vi "FPGA_I2C_Globals.vi"() -> ()   [LabVIEW 2020]
doc: "Stores configuration information for the I2C engine to be used by the top-level FPGA VI."
uses:
  Controls/FPGA I2C_Cmd.ctl
panel:
  in  "I2C_Address":u16
  in  "I2C_Bytes to Write":u16=1
  in  "I2C_Bytes to Read":u16=1
  in  "I2C_Wait Time/2":u32
  in  "I2C_Wait Time":u32
  in  "I2C_Cmd":T1=enum."Configure"
  out "I2C_Done":bool
  out "I2C_Start":bool
  in  "I2C_Port":u8
  # "Write Port, Address, Data (Write), Number of Bytes (Read) or Both"
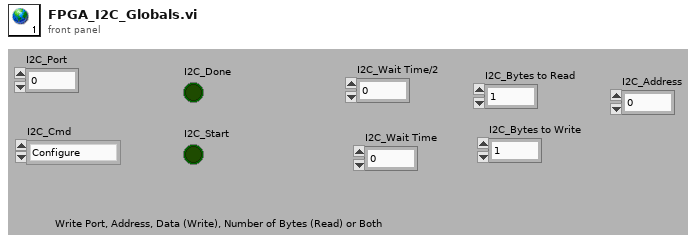
[diagram p1: front panel]
types:
  T1 = typedef "FPGA I2C_Cmd.ctl" = enum8{"Idle", "Write I2C", "Read I2C", "Write & Read I2C", "Configure"}
diagram:
